vi "LvMPDC_CMD_Open.vi"(6 "timeout_ms":i32=25000, 8 "error in (no error)":errorcluster, 10 "Port":u16=6600, 11 "Server":string) -> (0 "error out":errorcluster, 3 "Connect ID out":refnum<k5>)   [LabVIEW 2012]
panel:
  out "Reply":string
  # "LvMPDC:: Open - Connect MPDServer"
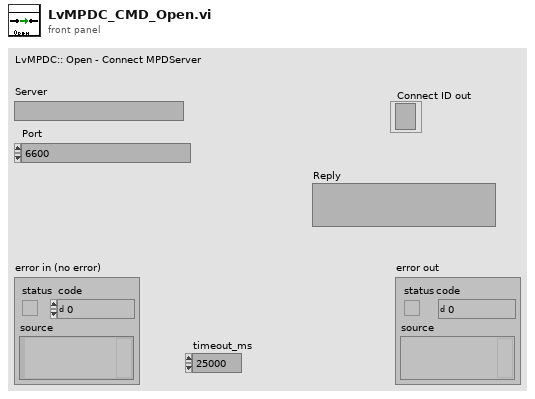
[diagram p1: front panel]
types:
  T1 = enum16{"Standard", "Buffered", "CRLF", "Immediate"}
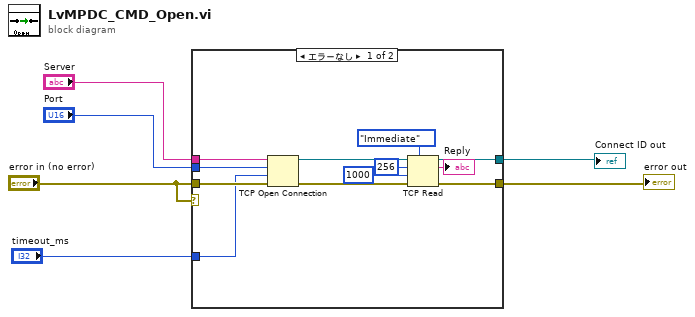
[diagram p0: block diagram]
diagram:
  n1 = case shown="エラーなし" "error in (no error)" {
    tunnel: "error in (no error)" -> [w18 w19]
    tunnel: [w10 _] -> w6
    tunnel: [w11 w19] -> w5
    tunnel: "timeout_ms" -> [w17 _]
    tunnel: "Port" -> [w16 _]
    tunnel: "Server" -> [w15 _]
    frame No Error {
      n2 = TCP Open Connection(address=w15, remote port or service name=w16, timeout ms (60000)=w17, error in (no error)=w18) -> (connection ID=w13:refnum<k5>, error out=w12:errorcluster)  [unwired: 1 in]
      n3 = TCP Read(connection ID=w13, bytes to read=256 ("読み取りバイト数"), error in (no error)=w12, 7:T1."Immediate" ("モード（標準）"), 9:1000 ("タイムアウト（ms）（25000）")) -> (connection ID out=w10:refnum<k5>, data out=→"Reply":string, error out=w11:errorcluster)
    }
    frame Error {
    }
  }
  "Connect ID out" <- w6
  "error out" <- w5
